vi "Open.vi"(8 "error in (no error)":errorcluster, 11 "Read CorVue in":refnum<class "Read CorVue.lvclass">) -> (0 "error out":errorcluster, 3 "Read CorVue out":refnum<class "Read CorVue.lvclass">)   [LabVIEW 2014, in "Read CorVue.lvclass"]
uses:
  Read CorVue.lvclass
  BScan.ctl
  <vilib>/Utility/file.llb/Read From Spreadsheet File (DBL).vi
  Read.lvclass
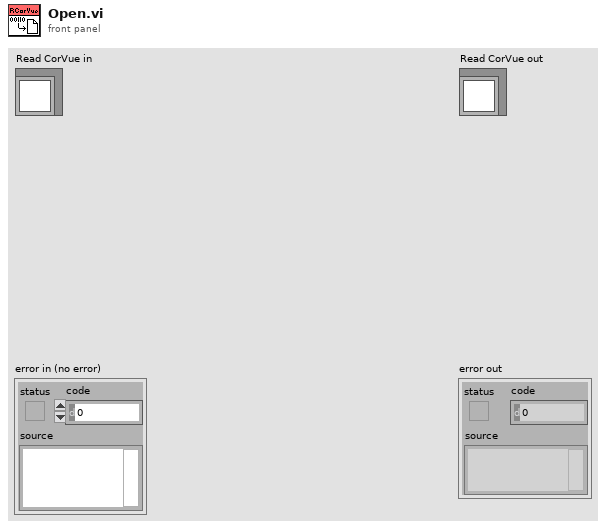
[diagram p1: front panel]
types:
  T1 = typedef "Read.lvclass/BScan.ctl" = cluster{"Points Per A-Scan":dbl, "A-Scans per B-Scan":dbl}
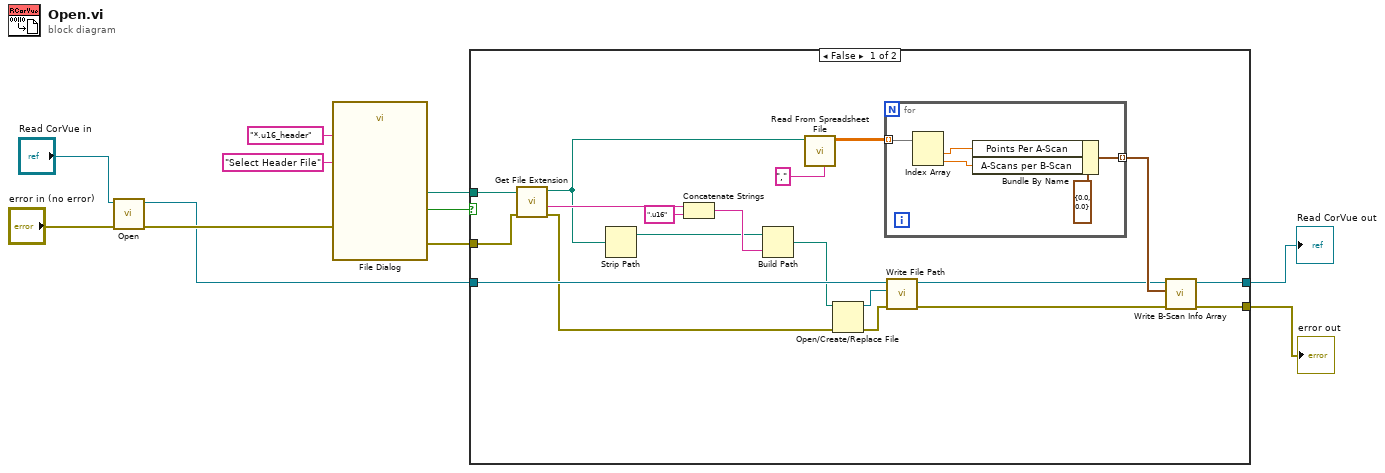
[diagram p0: block diagram]
diagram:
  n1 = call-parent "Open.vi"("error in (no error)"="error in (no error)", "Read in"="Read CorVue in") -> ("error out"=w7:errorcluster, "Read out"=w3:refnum<class "Read CorVue.lvclass">)  [unwired: 8 in]
  n2 = call "File Dialog"("prompt"="Select Header File", "error in"=w7, "pattern (all files)"="*.u16_header") -> ("selected path"=w6:path, "cancelled"=w5:bool, "error out"=w4:errorcluster)  [unwired: 9 in, 1 out]
  n3 = case shown="False" w5 {
    tunnel: w6 -> [w30 _]
    tunnel: w4 -> [w29 w37]
    tunnel: w3 -> [w21 w36]
    tunnel: [w18 w36] -> w2
    tunnel: [w17 w37] -> w1
    frame False {
      n4 = call <vilib>:"Get File Extension.vi"("error in (no error)"=w29, "file"=w30) -> ("error out"=w13:errorcluster, "filename without extension"=w28:string, "dup file"=w24:path)  [unwired: 6 in, 1 out]
      n5 = Strip Path(path=w24) -> (stripped path=w25:path)  [unwired: 1 out]
      n6 = Concatenate Strings(w28, ".u16" ("string")) -> (w26:string)
      n7 = Build Path(base path=w25, name or relative path=w26) -> (appended path=w15:path)
      n8 = call-poly <vilib>:"Read From Spreadsheet File.vi"("delimiter (\\t)"="," ("delimiter (\\t)"), "file path (dialog if empty)"=w24) -> ("all rows"=w22:dbl[][])  [unwired: 5 in, 4 out]
      n9 = Open/Create/Replace File(file path (use dialog)=w15, error in=w13) -> (refnum out=w14:refnum<file>, error out=w12:errorcluster)  [unwired: 4 in, 1 out]
      n10 = for {
        tunnel: w22 -> [w35] mode=indexing
        tunnel: [w31] -> w19 mode=indexing
        n11 = Index Array(array=w35) -> (element #1=w33:dbl, element #2=w32:dbl)  [unwired: 2 in]
        n12 = Bundle By Name(cluster=T1 {"Points Per A-Scan"=0.0, "A-Scans per B-Scan"=0.0} ("B-Scan"), "Points Per A-Scan"=w33, "A-Scans per B-Scan"=w32) -> (w31:T1)
      }
      n13 = call-dynamic "Write File Path.vi"("error in (no error)"=w12, "File Ref"=w14, "Read in"=w21) -> ("error out"=w20:errorcluster, "Read out"=w16:refnum<class "Read CorVue.lvclass">)  [unwired: 7 in]
      n14 = call-dynamic "Write B-Scan Info Array.vi"("error in (no error)"=w20, "B-Scan Info Array"=w19, "Read in"=w16) -> ("error out"=w17:errorcluster, "Read out"=w18:refnum<class "Read CorVue.lvclass">)  [unwired: 7 in]
    }
    frame True {
    }
  }
  "error out" <- w1
  "Read CorVue out" <- w2
